vi "Load FIFO U64.vi"(8 "error in (no error)":errorcluster, 9 "Data":u64[](array[numeric]), 10 "Base Path":string, 11 "FPGA Session In":refnum<class "FPGA Interface Base.lvclass">) -> (0 "error out":errorcluster, 3 "FPGA Session Out":refnum<class "FPGA Interface Base.lvclass">)   [LabVIEW 2011, in "Engine Sim RT.lvlib"]
uses:
  Engine Sim RT.lvlib
  <userlib>/_FPGA Interface Advanced Tools/FPGA Interface Base/FPGA Interface Base.lvclass
  <userlib>/_FPGA Interface Advanced Tools/FPGA Interface Base/FPGA Write By Name - Boolean.vi
  <userlib>/_FPGA Interface Advanced Tools/FPGA Interface Base/FPGA Write By Name - U64.vi
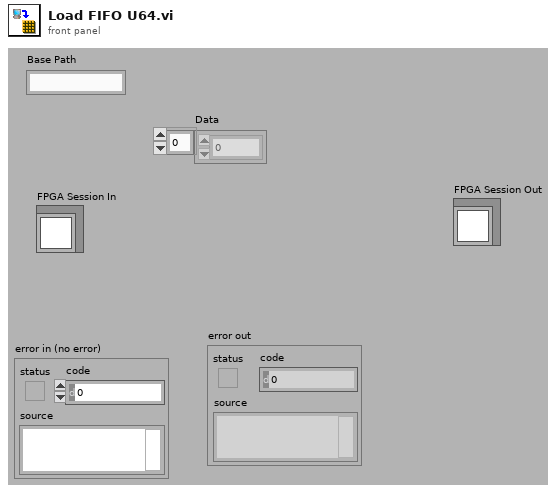
[diagram p1: front panel]
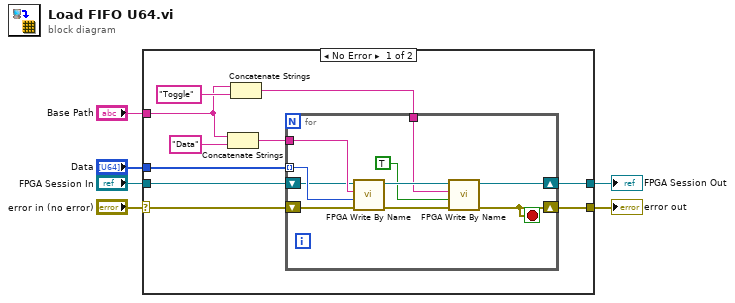
[diagram p0: block diagram]
diagram:
  n1 = case shown="No Error" "error in (no error)" {
    selector: "error in (no error)" -> [w15 w28]
    tunnel: [w16 w28] -> w6
    tunnel: [w11 w27] -> w4
    tunnel: "FPGA Session In" -> [w14 w27]
    tunnel: "Base Path" -> [w8 _]
    tunnel: "Data" -> [w7 _]
    frame No Error {
      n2 = Concatenate Strings(w8, "Data" ("string")) -> (w13:string)
      n3 = Concatenate Strings(w8, "Toggle" ("string")) -> (w12:string)
      n4 = for {
        shift-right: [w20] -> w16
        shift-left: w15 -> [w18]
        tunnel: w7 -> [w25] mode=indexing
        tunnel: w13 -> [w26]
        tunnel: w12 -> [w22]
        shift-right: [w19] -> w11
        shift-left: w14 -> [w17]
        stop <- w20 stop-if-true
        n5 = call-poly <userlib>:"FPGA Write By Name.vi"("error in (no error)"=w18, "Value"=w25, "Control"=w26, "FPGA Session In"=w17) -> ("error out"=w21:errorcluster, "FPGA Session Out"=w24:refnum<class "FPGA Interface Base.lvclass">)  [unwired: 6 in]
        n6 = call-poly <userlib>:"FPGA Write By Name.vi"("error in (no error)"=w21, "Value"=TRUE, "Control"=w22, "FPGA Session In"=w24) -> ("error out"=w20:errorcluster, "FPGA Session Out"=w19:refnum<class "FPGA Interface Base.lvclass">)  [unwired: 6 in]
      }
    }
    frame Error {
    }
  }
  "error out" <- w6
  "FPGA Session Out" <- w4
